vi "Setup UI.vi"(8 "error in (no error)":errorcluster, 10 "Set UI to input? (F)":bool, 11 "Anritsu Optical Power Meter  in":refnum<class "Anritsu Optical Power Meter .lvclass">) -> (0 "error out":errorcluster, 3 "Anritsu Optical Power Meter  out":refnum<class "Anritsu Optical Power Meter .lvclass">)   [LabVIEW 2012, in "Anritsu Optical Power Meter .lvclass"]
uses:
  Anritsu Optical Power Meter .lvclass
  Anritsu Power Meter/Public/Averaging control.ctl
  Anritsu Power Meter/Public/Auto Range control.ctl
  Anritsu Power Meter/Public/Display control.ctl
  Anritsu Optical Power Meter .lvclass/Anritsu Optical Power Meter .ctl
  Utility Classes/Readable/Readable.lvclass
panel:
  in  "Set":bool
  in  "Units":T1
  in  "Calibration Factor":dbl=-26.67
  in  "Auto Ranging?":T2
  in  "Averaging":T3
  # "Anritsu Setup"
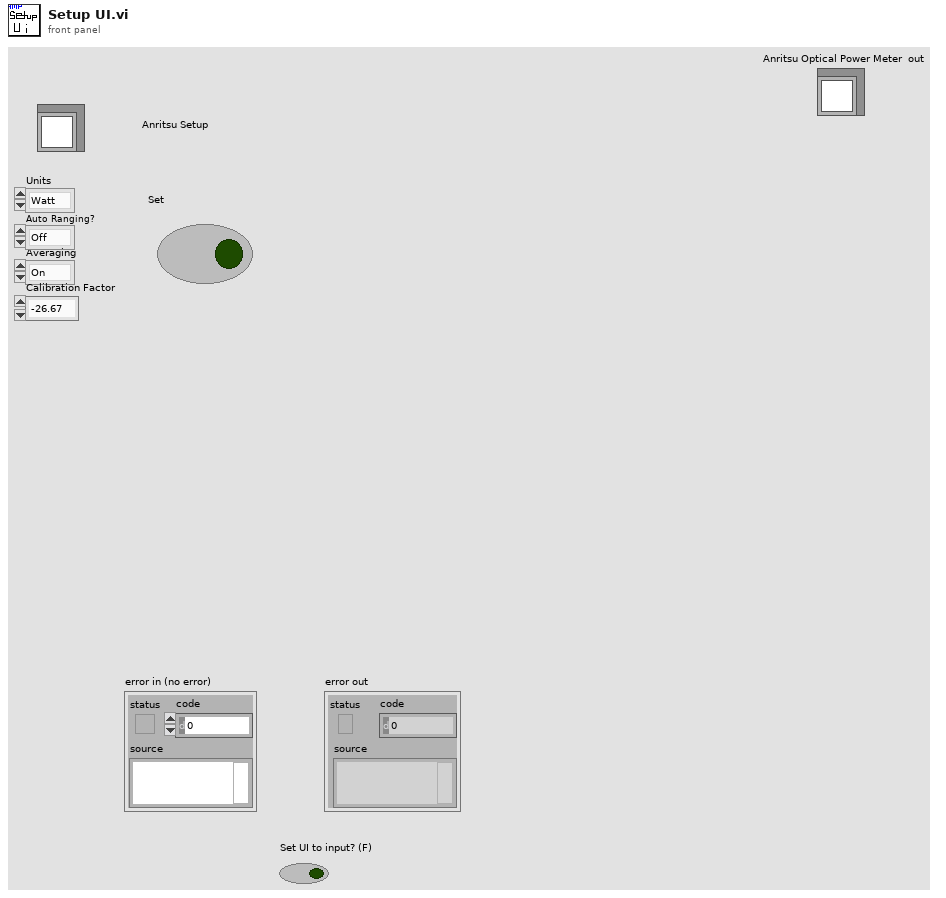
[diagram p1: front panel]
types:
  T1 = typedef "Display control.ctl" = enum16{"Watt", "dBm", "dB (REL)"}
  T2 = typedef "Auto Range control.ctl" = enum16{"Off", "On"}
  T3 = typedef "Averaging control.ctl" = enum16{"On", "Off"}
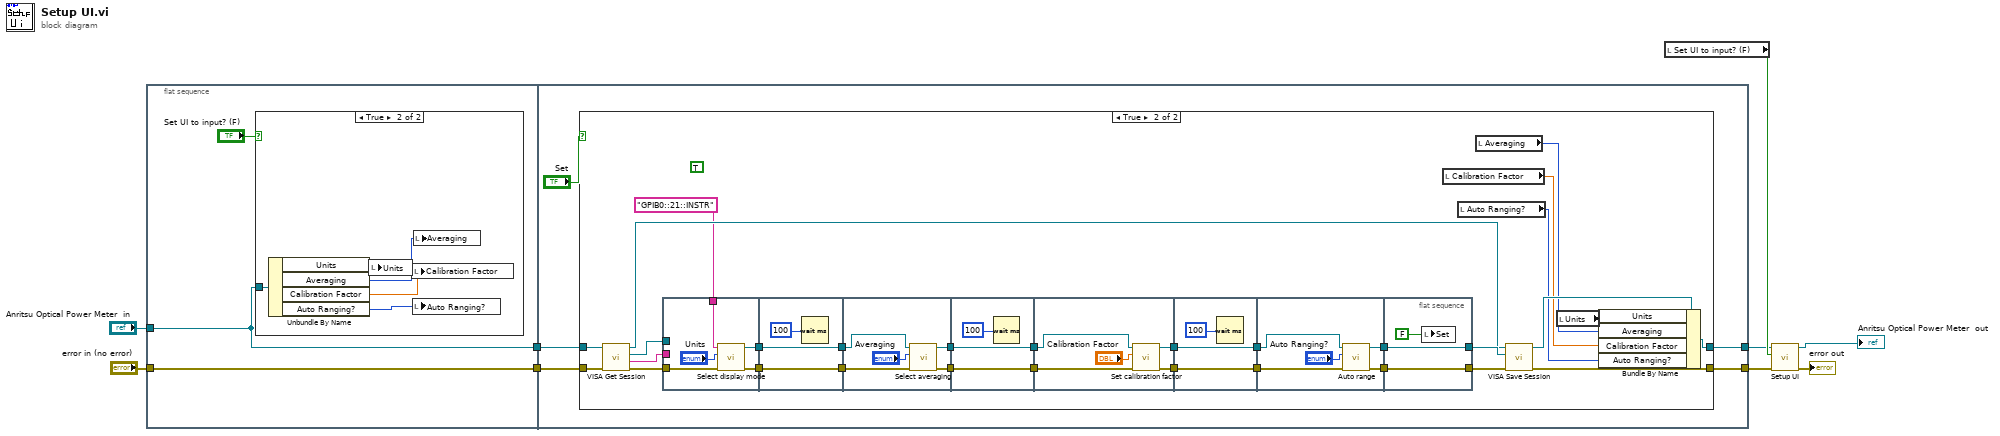
[diagram p0: block diagram]
diagram:
  n1 = flat-sequence {
    tunnel: "Anritsu Optical Power Meter  in" -> [w11]
    tunnel: [w11] -> w9
    tunnel: "error in (no error)" -> [w10]
    tunnel: [w10] -> w7
    tunnel: w9 -> [w22]
    tunnel: w7 -> [w21]
    tunnel: [w20] -> w5
    tunnel: [w19] -> w4
    frame #0 {
      n2 = case shown="True" "Set UI to input? (F)" {
        tunnel: w11 -> [_ w17]
        frame False {
        }
        frame True {
          n3 = Unbundle By Name(w17) -> ("Units"=w16:T1, "Averaging"=w15:T3, "Calibration Factor"=w13:dbl, "Auto Ranging?"=w14:T2)
          n4 = local write "Units"(w16) -> ()
          n5 = local write "Calibration Factor"(w13) -> ()
          n6 = local write "Auto Ranging?"(w14) -> ()
          n7 = local write "Averaging"(w15) -> ()
        }
      }
    }
    frame #1 {
      n8 = case shown="True" "Set" {
        tunnel: w22 -> [w24 w36]
        tunnel: w21 -> [w23 w54]
        tunnel: [w24 w33] -> w20
        tunnel: [w23 w35] -> w19
        frame False {
        }
        frame True {
          (unwired) TRUE
          n9 = call-dynamic "VISA Get Session.vi"("error in (no error)"=w54, "Instrument.lvclass in"=w36) -> ("error out"=w53:errorcluster, "GPIB string"=w25:string, "VISA Resource Name"=w27:refnum<visa-resource-name>, "Instrument.lvclass out"=w34:refnum<class "Anritsu Optical Power Meter .lvclass">)  [unwired: 6 in]
          n10 = flat-sequence {
            tunnel: w53 -> [w58]
            tunnel: [w57] -> w52
            tunnel: [w56] -> w51
            tunnel: w27 -> [_]
            tunnel: "GPIB0::21::INSTR" -> [w55]
            tunnel: w25 -> [_]
            tunnel: w52 -> [w60]
            tunnel: w51 -> [w61]
            tunnel: [w61] -> w50
            tunnel: [w60] -> w49
            tunnel: w50 -> [w65]
            tunnel: w49 -> [w66]
            tunnel: [w64] -> w48
            tunnel: [w63] -> w47
            tunnel: w48 -> [w69]
            tunnel: w47 -> [w68]
            tunnel: [w69] -> w46
            tunnel: [w68] -> w45
            tunnel: w46 -> [w74]
            tunnel: w45 -> [w73]
            tunnel: [w72] -> w44
            tunnel: [w71] -> w43
            tunnel: w44 -> [w78]
            tunnel: w43 -> [w77]
            tunnel: [w78] -> w42
            tunnel: [w77] -> w41
            tunnel: w42 -> [w82]
            tunnel: w41 -> [w81]
            tunnel: [w80] -> w40
            tunnel: [w79] -> w39
            tunnel: w40 -> [w84]
            tunnel: w39 -> [w85]
            tunnel: [w85] -> w38
            tunnel: [w84] -> w37
            frame #0 {
              n11 = call "Select display mode.vi"("error in (no error)"=w58, "Display"="Units", "VISA resource name"=w55) -> ("error out"=w56:errorcluster, "VISA resource name out"=w57:refnum<visa-resource-name>)  [unwired: 7 in]
            }
            frame #1 {
              n12 = Wait (ms)(milliseconds to wait=u32 100) -> ()  [unwired: 1 out]
            }
            frame #2 {
              n13 = call "Select averaging.vi"("error in (no error)"=w65, "Averaging"="Averaging", "VISA resource name"=w66) -> ("error out"=w63:errorcluster, "VISA resource name out"=w64:refnum<visa-resource-name>)  [unwired: 7 in]
            }
            frame #3 {
              n14 = Wait (ms)(milliseconds to wait=u32 100) -> ()  [unwired: 1 out]
            }
            frame #4 {
              n15 = call "Set calibration factor.vi"("error in (no error)"=w73, "Calibration Factor"="Calibration Factor", "VISA resource name"=w74) -> ("error out"=w71:errorcluster, "VISA resource name out"=w72:refnum<visa-resource-name>)  [unwired: 7 in]
            }
            frame #5 {
              n16 = Wait (ms)(milliseconds to wait=u32 100) -> ()  [unwired: 1 out]
            }
            frame #6 {
              n17 = call "Auto range.vi"("error in (no error)"=w81, "Auto Ranging?"="Auto Ranging?", "VISA resource name"=w82) -> ("error out"=w80:errorcluster, "VISA resource name out"=w79:refnum<visa-resource-name>)  [unwired: 7 in]
            }
            frame #7 {
              n18 = local write "Set"(FALSE) -> ()
            }
          }
          n19 = local read "Calibration Factor"() -> (w29:dbl)
          n20 = local read "Auto Ranging?"() -> (w30:T2)
          n21 = local read "Averaging"() -> (w31:T3)
          n22 = call-dynamic "VISA Save Session.vi"("error in (no error)"=w37, "VISA Resource Name"=w38, "Instrument.lvclass in"=w34) -> ("error out"=w35:errorcluster, "Instrument.lvclass out"=w32:refnum<class "Anritsu Optical Power Meter .lvclass">)  [unwired: 7 in]
          n23 = local read "Units"() -> (w28:T1)
          n24 = Bundle By Name(cluster=w32, "Units"=w28, "Averaging"=w31, "Calibration Factor"=w29, "Auto Ranging?"=w30) -> (w33:refnum<class "Anritsu Optical Power Meter .lvclass">)
        }
      }
    }
  }
  n25 = local read "Set UI to input? (F)"() -> (w6:bool)
  n26 = call-parent "Setup UI.vi"("error in (no error)"=w4, "Set UI to input? (F)"=w6, "Instrument in"=w5) -> ("error out"=→"error out":errorcluster, "Instrument out"=→"Anritsu Optical Power Meter  out":refnum<class "Anritsu Optical Power Meter .lvclass">)  [unwired: 7 in]
